vi "Assert Collection Equivalent.vi"(5 "Expected":variant, 7 "Message (\"\")":string, 8 "error in (no error)":errorcluster, 10 "Collection":variant) -> (0 "error out":errorcluster)   [LabVIEW 2017, in "Transparent Assertions.lvlib"]
doc: "Asserts that two collections (arrays, sets, or maps) are equivalent. Returns an error if the assertion fails, and optionally appends a custom message to the error.\n\nCollections are considered equivalent if they contain the same elements, regardless of order.\n\nFor maps, the values are compared for equivalence."
uses:
  Transparent Assertions.lvlib
  Collection Is Equivalent/Collection Is Equivalent.lvclass
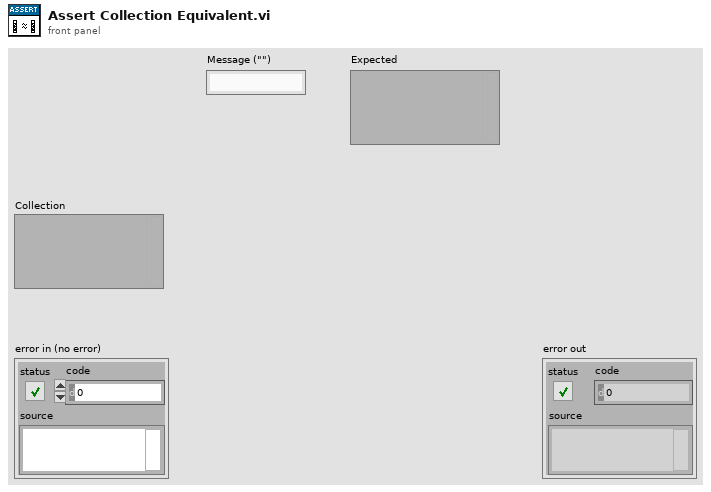
[diagram p1: front panel]
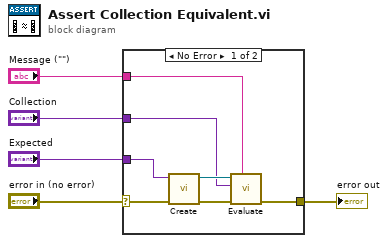
[diagram p0: block diagram]
diagram:
  n1 = case shown="No Error" "error in (no error)" {
    selector: "error in (no error)" -> [w8 w13]
    tunnel: [w12 w13] -> w5
    tunnel: "Expected" -> [w6 _]
    tunnel: "Message (\"\")" -> [w11 _]
    tunnel: "Collection" -> [w7 _]
    frame No Error {
      n2 = call "Create.vi"("error in (no error)"=w8, "Other"=w6) -> ("error out"=w10:errorcluster, "Collection Is Equivalent"=w9:refnum<class "Collection Is Equivalent.lvclass">)  [unwired: 8 in]
      n3 = call-dynamic "Evaluate.vi"("Message (\"\")"=w11, "error in (no error)"=w10, "Actual"=w7, "Constraint in"=w9) -> ("error out"=w12:errorcluster)  [unwired: 6 in, 1 out]
    }
    frame Error {
    }
  }
  "error out" <- w5
